vi "SLSC Convert Items - Variant to String.vi"(0 "Datatype":string, 1 "format string":string="%#_12g", 5 "value":variant, 7 "min":variant, 9 "max":variant, 11 "reset value":variant, 12 "Enum string":cluster{"name":string, "enum":string}[](array[cluster])) -> (3 "string data reset value":string, 4 "Output data type":string, 6 "string data value":string, 8 "string min":string, 10 "string max":string, 13 "Option":string, 14 "enum_range":string)   [LabVIEW 2019, in "SLSC Tree Control.lvlib"]
doc: "Converts all of the item elements from variant into strings."
uses:
  SLSC Tree Control.lvlib
  <vilib>/Utility/Data Type/Type Definitions/Data Type.ctl
  <vilib>/regexp/Match Regular Expression.xnode
  <vilib>/Utility/Data Type/NI_Data Type.lvlib
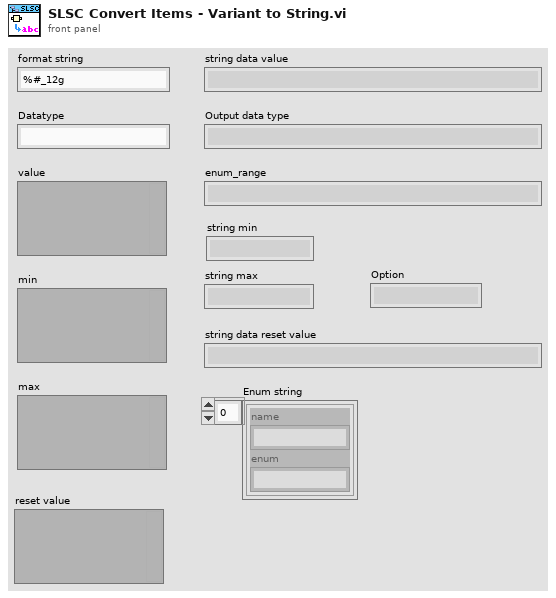
[diagram p1: front panel]
types:
  T1 = typedef "NI_Data Type.lvlib/Data Type.ctl" = enum8{"Invalid Type", "Void", "I8", "I16", "I32", "I64", "U8", "U16", "U32", "U64", "Single Float", "Double Float", "Extended Float", "Single Complex", "Double Complex", "Extended Complex", "Enum U8", "Enum U16", "Enum U32", "Enum U64", "Single Float With Unit", "Double Float With Unit", "Extended Float With Unit", "Single Complex with Unit", "Double Complex with Unit", "Extended Complex with Unit", "Boolean", "String", "Path", "Picture", "Tag", "Array", "Cluster", "Variant", "LV Variant", "Waveform", "Timestamp", "Digital Waveform", "Digital Data", "ExpressData", "Refnum", "External Data", "VI", "Poly VI", "LabVIEW Class Instance", "Fixed Point", "Set Collection", "Map Collection"}
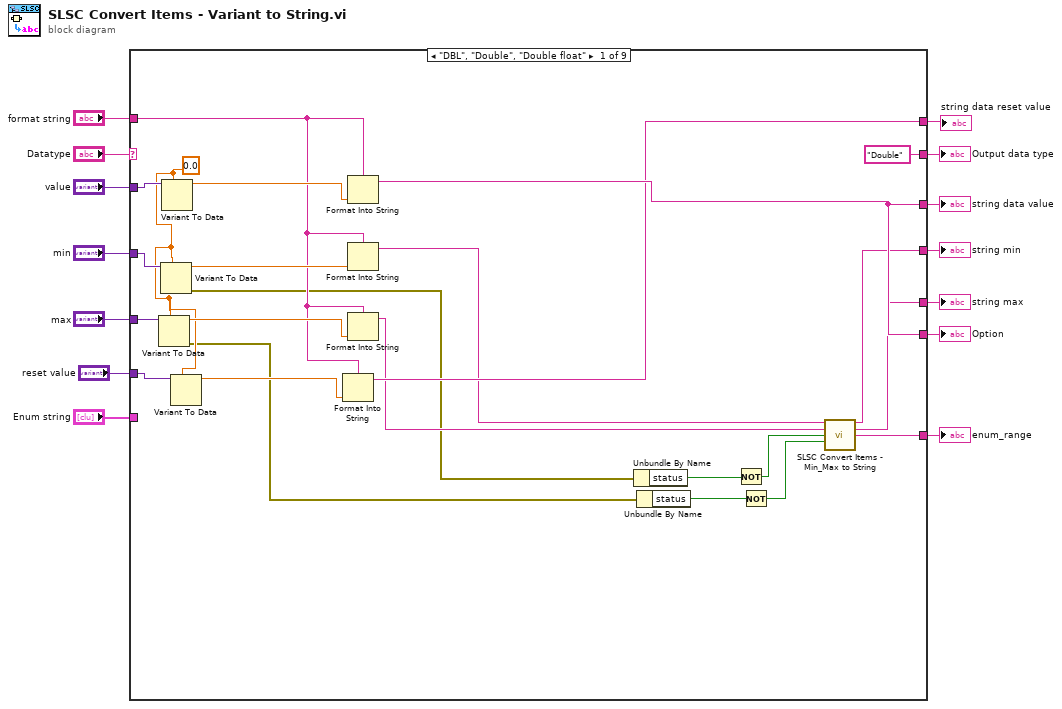
[diagram p0: block diagram]
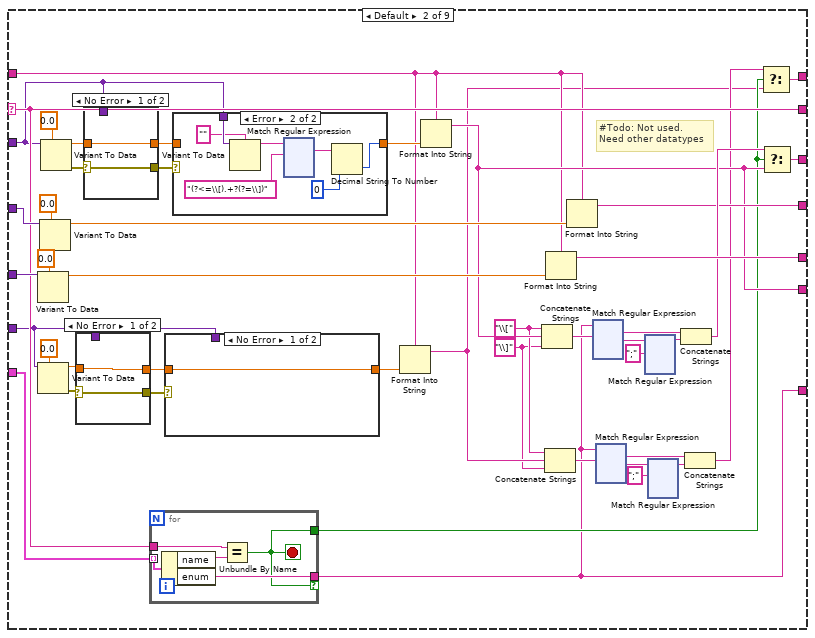
[diagram p2: hidden frame]
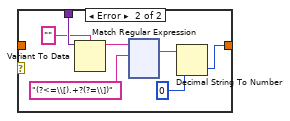
[diagram p3: hidden frame]
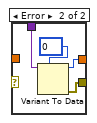
[diagram p4: hidden frame]
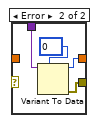
[diagram p6: hidden frame]
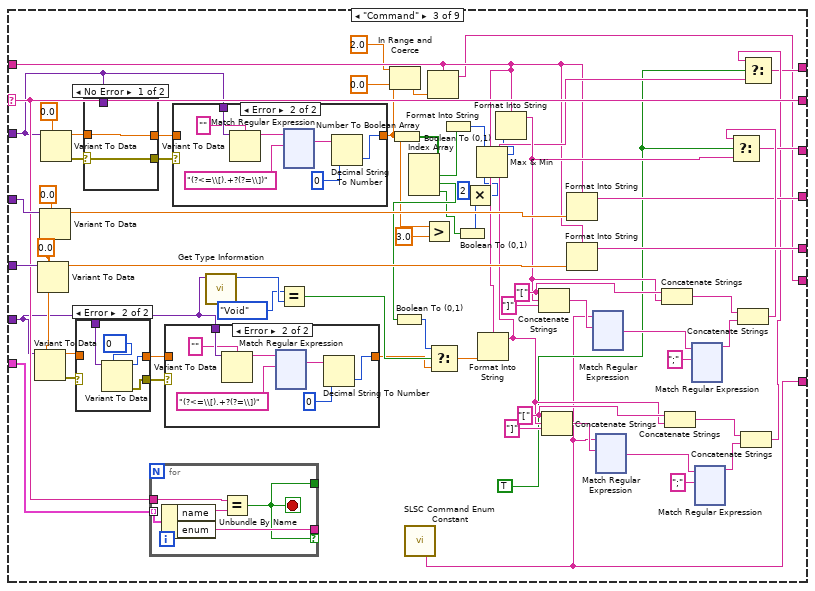
[diagram p7: hidden frame]
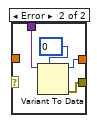
[diagram p11: hidden frame]
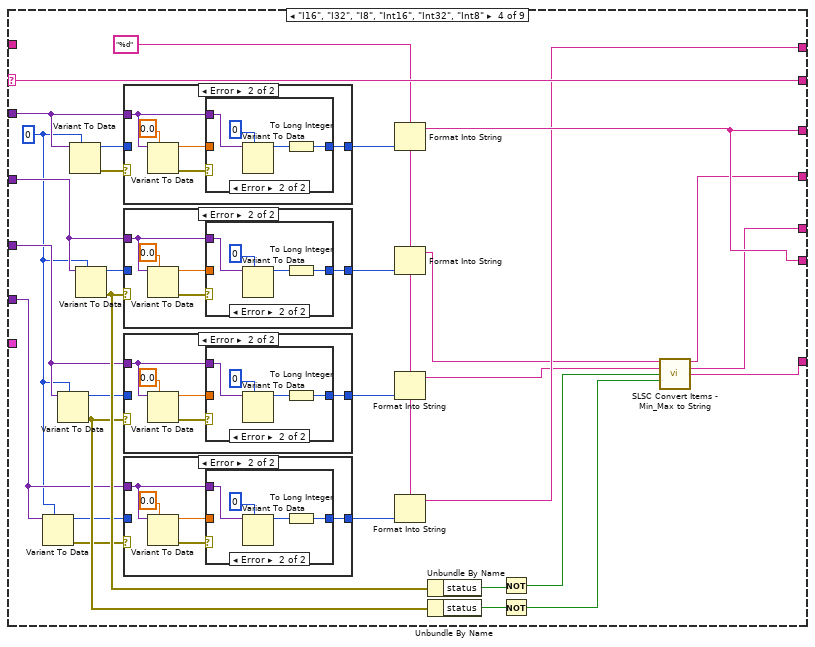
[diagram p12: hidden frame]
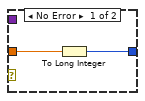
[diagram p14: hidden frame]
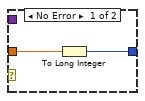
[diagram p16: hidden frame]
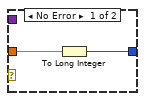
[diagram p18: hidden frame]
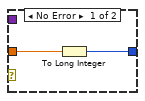
[diagram p20: hidden frame]
diagram:
  n1 = case shown="\"DBL\", \"Double\", \"Double float\"" "Datatype" {
    selector: "Datatype" -> [_ w75 w857 w1612 w1690 w1764 w1872 w1970 w2017]
    tunnel: "value" -> [w38 w63 w842 w1597 w1675 w1752 w1860 w1966 w2016]
    tunnel: [w32 w69 w848 w1611 w1689 w1763 w1871 w1971 w2015] -> w3
    tunnel: ["Double" w75 w857 w1612 w1690 w1764 w1872 w1970 w2017] -> w10
    tunnel: "min" -> [w36 w81 w863 w1595 w1673 w1745 w1857 _ _]
    tunnel: "max" -> [w35 w80 w862 w1591 w1669 w1746 w1853 _ _]
    tunnel: [w17 w66 w845 w1602 w1680 w1756 w1864 _ _] -> w6
    tunnel: [w16 w77 w859 w1601 w1679 w1755 w1863 _ _] -> w5
    tunnel: "format string" -> [w27 w53 w813 _ _ _ _ _ _]
    tunnel: "Enum string" -> [_ w76 w858 _ _ _ _ _ _]
    tunnel: [w18 w44 w816 w1603 w1681 w1757 w1865 _ _] -> w14
    tunnel: [w32 w65 w812 w1611 w1689 w1763 w1871 w1967 _] -> w4
    tunnel: "reset value" -> [w31 w54 w821 w1587 w1665 w1747 w1848 w1959 w2013]
    tunnel: [w28 w45 w826 w1610 w1688 w1762 w1870 w1955 w2012] -> w1
    frame "DBL", "Double", "Double float" {
      w30 = 0.0
      n2 = Variant To Data(type=w30, Variant=w35) -> (data=w33:dbl, error out=w23:errorcluster)  [unwired: 1 in]
      n3 = Variant To Data(type=w30, Variant=w36) -> (data=w34:dbl, error out=w24:errorcluster)  [unwired: 1 in]
      n4 = Variant To Data(type=w30, Variant=w38) -> (data=w37:dbl)  [unwired: 1 in, 1 out]
      n5 = Variant To Data(type=w30, Variant=w31) -> (data=w29:dbl)  [unwired: 1 in, 1 out]
      n6 = Format Into String(format string=w27, w29) -> (resulting string=w28:string)  [unwired: 2 in, 1 out]
      n7 = Format Into String(format string=w27, w37) -> (resulting string=w32:string)  [unwired: 2 in, 1 out]
      n8 = Format Into String(format string=w27, w34) -> (resulting string=w26:string)  [unwired: 2 in, 1 out]
      n9 = Format Into String(format string=w27, w33) -> (resulting string=w25:string)  [unwired: 2 in, 1 out]
      n10 = Unbundle By Name(w24) -> ("status"=w21:bool)
      n11 = Unbundle By Name(w23) -> ("status"=w22:bool)
      n12 = Not(x=w21) -> (.not. x?=w19:bool)
      n13 = Not(x=w22) -> (.not. x?=w20:bool)
      n14 = call "SLSC Convert Items - Min_Max to String.vi"("minimum"=w26, "maximum"=w25, "min?"=w19, "max?"=w20) -> ("minimum out"=w17:string, "maximum out"=w16:string, "minmax string"=w18:string)  [unwired: 9 in]
    }
    frame Default {
      w42 = "\\]" ("string")
      w43 = "\\[" ("string")
      # "#Todo: Not used.\nNeed other datatypes"
      n15 = Variant To Data(type=0.0, Variant=w80) -> (data=w78:dbl)  [unwired: 1 in, 1 out]
      n16 = Variant To Data(type=0.0, Variant=w54) -> (data=w56:dbl, error out=w57:errorcluster)  [unwired: 1 in]
      n17 = Variant To Data(type=0.0, Variant=w81) -> (data=w79:dbl)  [unwired: 1 in, 1 out]
      n18 = Variant To Data(type=0.0, Variant=w63) -> (data=w67:dbl, error out=w68:errorcluster)  [unwired: 1 in]
      n19 = case shown="No Error" w57 {
        selector: w57 -> [w434 _]
        tunnel: w54 -> [_ w439]
        tunnel: [w435 w438] -> w58
        tunnel: w56 -> [w435 _]
        tunnel: [w434 w436] -> w59
        frame No Error {
        }
        frame Error {
          w437 = u16 0 items=[""] ("Ring")
          n20 = Variant To Data(type=w437, Variant=w439) -> (data=w438:u16, error out=w436:errorcluster)  [unwired: 1 in]
        }
      }
      n21 = case shown="No Error" w68 {
        selector: w68 -> [w562 _]
        tunnel: w63 -> [_ w567]
        tunnel: [w563 w566] -> w64
        tunnel: w67 -> [w563 _]
        tunnel: [w562 w564] -> w62
        frame No Error {
        }
        frame Error {
          w565 = u16 0 items=[""] ("Ring")
          n22 = Variant To Data(type=w565, Variant=w567) -> (data=w566:u16, error out=w564:errorcluster)  [unwired: 1 in]
        }
      }
      n23 = for {
        tunnel: w76 -> [w800] mode=indexing
        tunnel: w75 -> [w798]
        tunnel: [w797] -> w44 if=w796
        tunnel: [w796] -> w48
        stop <- w796 stop-if-true
        n24 = Unbundle By Name(w800) -> ("name"=w799:string, "enum"=w797:string)
        n25 = Equal?(x=w798, y=w799) -> (x = y?=w796:bool)
      }
      n26 = case shown="No Error" w59 {
        tunnel: w54 -> [_ w319]
        tunnel: [w312 w313] -> w60
        tunnel: w58 -> [w312 _]
        frame No Error {
        }
        frame Error {
          n27 = Variant To Data(type="", Variant=w319) -> (data=w317:string)  [unwired: 1 in, 1 out]
          n28 = xnode "Match Regular Expression"("input string"=w317, "regular expression"="(?<=\\[).+?(?=\\])") -> ("whole match"=w315:string)  [unwired: 4 in, 4 out]
          n29 = Decimal String To Number(string=w315, default (0L)=0) -> (number=w313:i32)  [unwired: 1 in, 1 out]
        }
      }
      n30 = case shown="Error" w62 {
        tunnel: w63 -> [_ w447]
        tunnel: [w440 w441] -> w61
        tunnel: w64 -> [w440 _]
        frame No Error {
        }
        frame Error {
          n31 = Variant To Data(type="", Variant=w447) -> (data=w445:string)  [unwired: 1 in, 1 out]
          n32 = xnode "Match Regular Expression"("input string"=w445, "regular expression"="(?<=\\[).+?(?=\\])") -> ("whole match"=w443:string)  [unwired: 4 in, 4 out]
          n33 = Decimal String To Number(string=w443, default (0L)=0) -> (number=w441:i32)  [unwired: 1 in, 1 out]
        }
      }
      n34 = Format Into String(format string=w53, w60) -> (resulting string=w46:string)  [unwired: 2 in, 1 out]
      n35 = Format Into String(format string=w53, w61) -> (resulting string=w65:string)  [unwired: 2 in, 1 out]
      n36 = Concatenate Strings(w43, w65, w42) -> (w71:string)
      n37 = Concatenate Strings(w43, w46, w42) -> (w52:string)
      n38 = Format Into String(format string=w53, w78) -> (resulting string=w77:string)  [unwired: 2 in, 1 out]
      n39 = Format Into String(format string=w53, w79) -> (resulting string=w66:string)  [unwired: 2 in, 1 out]
      n40 = xnode "Match Regular Expression"("input string"=w44, "regular expression"=w71) -> ("whole match"=w41:string, "after match"=w74:string)  [unwired: 4 in, 3 out]
      n41 = xnode "Match Regular Expression"("input string"=w44, "regular expression"=w52) -> ("whole match"=w40:string, "after match"=w49:string)  [unwired: 4 in, 3 out]
      n42 = xnode "Match Regular Expression"("input string"=w74, "regular expression"=";") -> ("before match"=w72:string)  [unwired: 4 in, 4 out]
      n43 = xnode "Match Regular Expression"("input string"=w49, "regular expression"=";") -> ("before match"=w51:string)  [unwired: 4 in, 4 out]
      n44 = Concatenate Strings(w41, w72) -> (w70:string)
      n45 = Concatenate Strings(w40, w51) -> (w47:string)
      n46 = Select(t=w47, s=w48, f=w46) -> (s? t:f=w45:string)
      n47 = Select(t=w70, s=w48, f=w65) -> (s? t:f=w69:string)
    }
    frame "Command" {
      w825 = TRUE ("s")
      w834 = "[" ("string")
      w851 = "[" ("string")
      w836 = 0.0
      n48 = Variant To Data(type=w836, Variant=w821) -> (data=w837:dbl, error out=w838:errorcluster)  [unwired: 1 in]
      n49 = Variant To Data(type=w836, Variant=w862) -> (data=w860:dbl)  [unwired: 1 in, 1 out]
      n50 = Variant To Data(type=0.0, Variant=w863) -> (data=w861:dbl)  [unwired: 1 in, 1 out]
      n51 = Variant To Data(type=0.0, Variant=w842) -> (data=w846:dbl, error out=w847:errorcluster)  [unwired: 1 in]
      n52 = case shown="Error" w838 {
        selector: w838 -> [w1216 _]
        tunnel: w821 -> [_ w1221]
        tunnel: [w1217 w1220] -> w839
        tunnel: w837 -> [w1217 _]
        tunnel: [w1216 w1218] -> w840
        frame No Error {
        }
        frame Error {
          w1219 = u16 0 items=[""] ("Ring")
          n53 = Variant To Data(type=w1219, Variant=w1221) -> (data=w1220:u16, error out=w1218:errorcluster)  [unwired: 1 in]
        }
      }
      n54 = case shown="No Error" w847 {
        selector: w847 -> [w1344 _]
        tunnel: w842 -> [_ w1349]
        tunnel: [w1345 w1348] -> w843
        tunnel: w846 -> [w1345 _]
        tunnel: [w1344 w1346] -> w841
        frame No Error {
        }
        frame Error {
          w1347 = u16 0 items=[""] ("Ring")
          n55 = Variant To Data(type=w1347, Variant=w1349) -> (data=w1348:u16, error out=w1346:errorcluster)  [unwired: 1 in]
        }
      }
      n56 = for {
        tunnel: w858 -> [w1582] mode=indexing
        tunnel: w857 -> [w1580]
        tunnel: [w1579] -> _ if=w1578
        tunnel: [w1578] -> _
        stop <- w1578 stop-if-true
        n57 = Unbundle By Name(w1582) -> ("name"=w1581:string, "enum"=w1579:string)
        n58 = Equal?(x=w1580, y=w1581) -> (x = y?=w1578:bool)
      }
      n59 = case shown="Error" w840 {
        tunnel: w821 -> [_ w1101]
        tunnel: [w1094 w1095] -> w815
        tunnel: w839 -> [w1094 _]
        frame No Error {
        }
        frame Error {
          n60 = Variant To Data(type="", Variant=w1101) -> (data=w1099:string)  [unwired: 1 in, 1 out]
          n61 = xnode "Match Regular Expression"("input string"=w1099, "regular expression"="(?<=\\[).+?(?=\\])") -> ("whole match"=w1097:string)  [unwired: 4 in, 4 out]
          n62 = Decimal String To Number(string=w1097, default (0L)=0) -> (number=w1095:i32)  [unwired: 1 in, 1 out]
        }
      }
      n63 = case shown="Error" w841 {
        tunnel: w842 -> [_ w1229]
        tunnel: [w1222 w1223] -> w811
        tunnel: w843 -> [w1222 _]
        frame No Error {
        }
        frame Error {
          n64 = Variant To Data(type="", Variant=w1229) -> (data=w1227:string)  [unwired: 1 in, 1 out]
          n65 = xnode "Match Regular Expression"("input string"=w1227, "regular expression"="(?<=\\[).+?(?=\\])") -> ("whole match"=w1225:string)  [unwired: 4 in, 4 out]
          n66 = Decimal String To Number(string=w1225, default (0L)=0) -> (number=w1223:i32)  [unwired: 1 in, 1 out]
        }
      }
      n67 = call <vilib>:"Get Type Information.vi"("variant"=w821) -> ("type"=w820:T1)  [unwired: 6 in, 4 out]
      n68 = Equal?(x=Data_Type."Void", y=w820) -> (x = y?=w818:bool)
      n69 = In Range and Coerce(upper limit=2.0 ("x"), x=w811, lower limit=0.0 ("x")) -> (coerced(x)=w807:dbl)  [unwired: 1 out]
      n70 = Number To Boolean Array(number=w811) -> (Boolean array=w824:bool[])
      n71 = call "SLSC Command Enum Constant.vi"() -> ("string enums"=w816:string)  [unwired: 11 in, 4 out]
      n72 = Index Array(array=w824) -> (element #1=w823:bool, element #2=w822:bool, element #3=w804:bool)  [unwired: 3 in]
      n73 = Boolean To (0,1)(Boolean=w822) -> (0, 1=w817:i16)
      n74 = Greater?(x=w811, y=3.0) -> ()  [unwired: 1 out]
      n75 = Format Into String(format string=w813, w807) -> (resulting string=w812:string)  [unwired: 2 in, 1 out]
      n76 = Select(t=w817, s=w818, f=w815) -> (s? t:f=w814:dbl)
      n77 = Boolean To (0,1)(Boolean=w823) -> (0, 1=w802:i16)
      n78 = Boolean To (0,1)(Boolean=w804) -> (0, 1=w809:i16)
      n79 = Multiply(x=i16 2, y=w809) -> (x*y=w803:i16)
      n80 = Max & Min(x=w802, y=w803) -> (max(x,y)=w801:i16)  [unwired: 1 out]
      n81 = Format Into String(format string=w813, w814) -> (resulting string=w827:string)  [unwired: 2 in, 1 out]
      n82 = Format Into String(format string=w813, w801) -> (resulting string=w844:string)  [unwired: 2 in, 1 out]
      n83 = Concatenate Strings(w851, w844, "]" ("string")) -> (w852:string)
      n84 = Concatenate Strings(w834, w827, "]" ("string")) -> (w833:string)
      n85 = Format Into String(format string=w813, w861) -> (resulting string=w845:string)  [unwired: 2 in, 1 out]
      n86 = Format Into String(format string=w813, w860) -> (resulting string=w859:string)  [unwired: 2 in, 1 out]
      n87 = xnode "Match Regular Expression"("input string"=w816, "regular expression"=w852) -> ("after match"=w855:string)  [unwired: 4 in, 4 out]
      n88 = xnode "Match Regular Expression"("input string"=w816, "regular expression"=w833) -> ("after match"=w830:string)  [unwired: 4 in, 4 out]
      n89 = Concatenate Strings(w851, w844) -> (w850:string)
      n90 = Concatenate Strings(w834, w827) -> (w835:string)
      n91 = xnode "Match Regular Expression"("input string"=w855, "regular expression"=";") -> ("before match"=w853:string)  [unwired: 4 in, 4 out]
      n92 = xnode "Match Regular Expression"("input string"=w830, "regular expression"=";") -> ("before match"=w832:string)  [unwired: 4 in, 4 out]
      n93 = Concatenate Strings(w850, w853) -> (w849:string)
      n94 = Select(t=w849, s=w825, f=w844) -> (s? t:f=w848:string)
      n95 = Concatenate Strings(w835, w832) -> (w828:string)
      n96 = Select(t=w828, s=w825, f=w827) -> (s? t:f=w826:string)
    }
    frame "I16", "I32", "I8", "Int16", "Int32", "Int8" {
      w1583 = 0
      w1600 = "%d" ("format string")
      n97 = Variant To Data(type=w1583, Variant=w1587) -> (data=w1585:i32, error out=w1586:errorcluster)  [unwired: 1 in]
      n98 = Variant To Data(type=w1583, Variant=w1591) -> (data=w1588:i32, error out=w1589:errorcluster)  [unwired: 1 in]
      n99 = Variant To Data(type=w1583, Variant=w1597) -> (data=w1599:i32, error out=w1598:errorcluster)  [unwired: 1 in]
      n100 = Variant To Data(type=w1583, Variant=w1595) -> (data=w1594:i32, error out=w1593:errorcluster)  [unwired: 1 in]
      n101 = case shown="Error" w1598 {
        tunnel: [w1649 w1651] -> w1596
        tunnel: w1599 -> [w1649 _]
        tunnel: w1597 -> [_ w1653]
        frame No Error {
        }
        frame Error {
          n102 = Variant To Data(type=0.0, Variant=w1653) -> (data=w1650:dbl, error out=w1652:errorcluster)  [unwired: 1 in]
          n103 = case shown="Error" w1652 {
            tunnel: w1653 -> [_ w1659]
            tunnel: [w1655 w1657] -> w1651
            tunnel: w1650 -> [w1656 _]
            frame No Error {
              n104 = To Long Integer(number=w1656) -> (32bit integer=w1655:i32)
            }
            frame Error {
              n105 = Variant To Data(type=i16 0, Variant=w1659) -> (data=w1658:i16)  [unwired: 1 in, 1 out]
              n106 = To Long Integer(number=w1658) -> (32bit integer=w1657:i32)
            }
          }
        }
      }
      n107 = case shown="Error" w1593 {
        tunnel: [w1637 w1639] -> w1592
        tunnel: w1594 -> [w1637 _]
        tunnel: w1595 -> [_ w1641]
        frame No Error {
        }
        frame Error {
          n108 = Variant To Data(type=0.0, Variant=w1641) -> (data=w1638:dbl, error out=w1640:errorcluster)  [unwired: 1 in]
          n109 = case shown="Error" w1640 {
            tunnel: w1641 -> [_ w1647]
            tunnel: [w1643 w1645] -> w1639
            tunnel: w1638 -> [w1644 _]
            frame No Error {
              n110 = To Long Integer(number=w1644) -> (32bit integer=w1643:i32)
            }
            frame Error {
              n111 = Variant To Data(type=i16 0, Variant=w1647) -> (data=w1646:i16)  [unwired: 1 in, 1 out]
              n112 = To Long Integer(number=w1646) -> (32bit integer=w1645:i32)
            }
          }
        }
      }
      n113 = case shown="Error" w1589 {
        tunnel: [w1625 w1627] -> w1590
        tunnel: w1588 -> [w1625 _]
        tunnel: w1591 -> [_ w1629]
        frame No Error {
        }
        frame Error {
          n114 = Variant To Data(type=0.0, Variant=w1629) -> (data=w1626:dbl, error out=w1628:errorcluster)  [unwired: 1 in]
          n115 = case shown="Error" w1628 {
            tunnel: w1629 -> [_ w1635]
            tunnel: [w1631 w1633] -> w1627
            tunnel: w1626 -> [w1632 _]
            frame No Error {
              n116 = To Long Integer(number=w1632) -> (32bit integer=w1631:i32)
            }
            frame Error {
              n117 = Variant To Data(type=i16 0, Variant=w1635) -> (data=w1634:i16)  [unwired: 1 in, 1 out]
              n118 = To Long Integer(number=w1634) -> (32bit integer=w1633:i32)
            }
          }
        }
      }
      n119 = case shown="Error" w1586 {
        tunnel: [w1613 w1615] -> w1584
        tunnel: w1585 -> [w1613 _]
        tunnel: w1587 -> [_ w1617]
        frame No Error {
        }
        frame Error {
          n120 = Variant To Data(type=0.0, Variant=w1617) -> (data=w1614:dbl, error out=w1616:errorcluster)  [unwired: 1 in]
          n121 = case shown="Error" w1616 {
            tunnel: w1617 -> [_ w1623]
            tunnel: [w1619 w1621] -> w1615
            tunnel: w1614 -> [w1620 _]
            frame No Error {
              n122 = To Long Integer(number=w1620) -> (32bit integer=w1619:i32)
            }
            frame Error {
              n123 = Variant To Data(type=i16 0, Variant=w1623) -> (data=w1622:i16)  [unwired: 1 in, 1 out]
              n124 = To Long Integer(number=w1622) -> (32bit integer=w1621:i32)
            }
          }
        }
      }
      n125 = Format Into String(format string=w1600, w1596) -> (resulting string=w1611:string)  [unwired: 2 in, 1 out]
      n126 = Format Into String(format string=w1600, w1592) -> (resulting string=w1605:string)  [unwired: 2 in, 1 out]
      n127 = Format Into String(format string=w1600, w1590) -> (resulting string=w1604:string)  [unwired: 2 in, 1 out]
      n128 = Format Into String(format string=w1600, w1584) -> (resulting string=w1610:string)  [unwired: 2 in, 1 out]
      n129 = Unbundle By Name(w1593) -> ("status"=w1608:bool)
      n130 = Unbundle By Name(w1589) -> ("status"=w1609:bool)
      n131 = Not(x=w1608) -> (.not. x?=w1606:bool)
      n132 = Not(x=w1609) -> (.not. x?=w1607:bool)
      n133 = call "SLSC Convert Items - Min_Max to String.vi"("minimum"=w1605, "maximum"=w1604, "min?"=w1606, "max?"=w1607) -> ("minimum out"=w1602:string, "maximum out"=w1601:string, "minmax string"=w1603:string)  [unwired: 9 in]
    }
    frame "U16", "U32", "U8", "UInt16", "UInt32", "UInt8" {
      w1661 = u32 0
      w1678 = "%d" ("format string")
      n134 = Variant To Data(type=w1661, Variant=w1665) -> (data=w1663:u32, error out=w1664:errorcluster)  [unwired: 1 in]
      n135 = Variant To Data(type=w1661, Variant=w1669) -> (data=w1666:u32, error out=w1667:errorcluster)  [unwired: 1 in]
      n136 = Variant To Data(type=w1661, Variant=w1675) -> (data=w1677:u32, error out=w1676:errorcluster)  [unwired: 1 in]
      n137 = Variant To Data(type=w1661, Variant=w1673) -> (data=w1672:u32, error out=w1671:errorcluster)  [unwired: 1 in]
      n138 = case shown="Error" w1676 {
        tunnel: [w1727 w1729] -> w1674
        tunnel: w1677 -> [w1727 _]
        tunnel: w1675 -> [_ w1731]
        frame No Error {
        }
        frame Error {
          n139 = Variant To Data(type=0.0, Variant=w1731) -> (data=w1728:dbl, error out=w1730:errorcluster)  [unwired: 1 in]
          n140 = case shown="Error" w1730 {
            tunnel: w1731 -> [_ w1737]
            tunnel: [w1733 w1735] -> w1729
            tunnel: w1728 -> [w1734 _]
            frame No Error {
              n141 = To Long Integer(number=w1734) -> (32bit integer=w1733:i32)
            }
            frame Error {
              n142 = Variant To Data(type=u16 0, Variant=w1737) -> (data=w1736:u16)  [unwired: 1 in, 1 out]
              n143 = To Unsigned Long Integer(number=w1736) -> (unsigned 32bit integer=w1735:u32)
            }
          }
        }
      }
      n144 = case shown="Error" w1671 {
        tunnel: [w1715 w1717] -> w1670
        tunnel: w1672 -> [w1715 _]
        tunnel: w1673 -> [_ w1719]
        frame No Error {
        }
        frame Error {
          n145 = Variant To Data(type=0.0, Variant=w1719) -> (data=w1716:dbl, error out=w1718:errorcluster)  [unwired: 1 in]
          n146 = case shown="Error" w1718 {
            tunnel: w1719 -> [_ w1725]
            tunnel: [w1721 w1723] -> w1717
            tunnel: w1716 -> [w1722 _]
            frame No Error {
              n147 = To Long Integer(number=w1722) -> (32bit integer=w1721:i32)
            }
            frame Error {
              n148 = Variant To Data(type=u16 0, Variant=w1725) -> (data=w1724:u16)  [unwired: 1 in, 1 out]
              n149 = To Unsigned Long Integer(number=w1724) -> (unsigned 32bit integer=w1723:u32)
            }
          }
        }
      }
      n150 = case shown="Error" w1667 {
        tunnel: [w1703 w1705] -> w1668
        tunnel: w1666 -> [w1703 _]
        tunnel: w1669 -> [_ w1707]
        frame No Error {
        }
        frame Error {
          n151 = Variant To Data(type=0.0, Variant=w1707) -> (data=w1704:dbl, error out=w1706:errorcluster)  [unwired: 1 in]
          n152 = case shown="Error" w1706 {
            tunnel: w1707 -> [_ w1713]
            tunnel: [w1709 w1711] -> w1705
            tunnel: w1704 -> [w1710 _]
            frame No Error {
              n153 = To Long Integer(number=w1710) -> (32bit integer=w1709:i32)
            }
            frame Error {
              n154 = Variant To Data(type=u16 0, Variant=w1713) -> (data=w1712:u16)  [unwired: 1 in, 1 out]
              n155 = To Unsigned Long Integer(number=w1712) -> (unsigned 32bit integer=w1711:u32)
            }
          }
        }
      }
      n156 = case shown="Error" w1664 {
        tunnel: [w1691 w1693] -> w1662
        tunnel: w1663 -> [w1691 _]
        tunnel: w1665 -> [_ w1695]
        frame No Error {
        }
        frame Error {
          n157 = Variant To Data(type=0.0, Variant=w1695) -> (data=w1692:dbl, error out=w1694:errorcluster)  [unwired: 1 in]
          n158 = case shown="Error" w1694 {
            tunnel: w1695 -> [_ w1701]
            tunnel: [w1697 w1699] -> w1693
            tunnel: w1692 -> [w1698 _]
            frame No Error {
              n159 = To Long Integer(number=w1698) -> (32bit integer=w1697:i32)
            }
            frame Error {
              n160 = Variant To Data(type=u16 0, Variant=w1701) -> (data=w1700:u16)  [unwired: 1 in, 1 out]
              n161 = To Unsigned Long Integer(number=w1700) -> (unsigned 32bit integer=w1699:u32)
            }
          }
        }
      }
      n162 = Format Into String(format string=w1678, w1674) -> (resulting string=w1689:string)  [unwired: 2 in, 1 out]
      n163 = Format Into String(format string=w1678, w1670) -> (resulting string=w1683:string)  [unwired: 2 in, 1 out]
      n164 = Format Into String(format string=w1678, w1668) -> (resulting string=w1682:string)  [unwired: 2 in, 1 out]
      n165 = Format Into String(format string=w1678, w1662) -> (resulting string=w1688:string)  [unwired: 2 in, 1 out]
      n166 = Unbundle By Name(w1671) -> ("status"=w1686:bool)
      n167 = Unbundle By Name(w1667) -> ("status"=w1687:bool)
      n168 = Not(x=w1686) -> (.not. x?=w1684:bool)
      n169 = Not(x=w1687) -> (.not. x?=w1685:bool)
      n170 = call "SLSC Convert Items - Min_Max to String.vi"("minimum"=w1683, "maximum"=w1682, "min?"=w1684, "max?"=w1685) -> ("minimum out"=w1680:string, "maximum out"=w1679:string, "minmax string"=w1681:string)  [unwired: 9 in]
    }
    frame "U64", "Uint64" {
      w1739 = u64 0
      w1754 = "%d" ("format string")
      n171 = call <vilib>:"Get Type Information.vi"("variant"=w1752) -> ("type"=w1751:T1)  [unwired: 6 in, 4 out]
      n172 = call <vilib>:"Get Type Information.vi"("variant"=w1747) -> ("type"=w1748:T1)  [unwired: 6 in, 4 out]
      n173 = call <vilib>:"Get Type Information.vi"("variant"=w1745) -> ("type"=w1750:T1)  [unwired: 6 in, 4 out]
      n174 = call <vilib>:"Get Type Information.vi"("variant"=w1746) -> ("type"=w1749:T1)  [unwired: 6 in, 4 out]
      n175 = case shown="\"U32\"" w1751 {
        tunnel: [_ w1828 w1830 w1834 w1838 w1843] -> w1753
        tunnel: w1752 -> [_ w1829 w1833 w1837 w1841 w1845]
        tunnel: w1739 -> [_ w1827 _ _ _ w1842]
        frame "Invalid Type", "Void", Default {
        }
        frame "U64" {
          n176 = Variant To Data(type=w1827, Variant=w1829) -> (data=w1828:u64)  [unwired: 1 in, 1 out]
        }
        frame "U32" {
          n177 = Variant To Data(type=u32 0, Variant=w1833) -> (data=w1832:u32)  [unwired: 1 in, 1 out]
          n178 = To Unsigned Quad Integer(1:w1832) -> (0:w1830:u64)
        }
        frame "U16" {
          n179 = Variant To Data(type=u16 0, Variant=w1837) -> (data=w1836:u16)  [unwired: 1 in, 1 out]
          n180 = To Unsigned Quad Integer(1:w1836) -> (0:w1834:u64)
        }
        frame "U8" {
          n181 = Variant To Data(type=u8 0, Variant=w1841) -> (data=w1840:u8)  [unwired: 1 in, 1 out]
          n182 = To Unsigned Quad Integer(1:w1840) -> (0:w1838:u64)
        }
        frame "Double Float" {
          n183 = Variant To Data(type=0.0, Variant=w1845) -> (data=w1844:dbl)  [unwired: 1 in, 1 out]
          n184 = Type Cast(type=w1842, x=w1844) -> (*(type *) &x=w1843:u64)
        }
      }
      n185 = case shown="\"Double Float\"" w1748 {
        tunnel: [_ w1766 w1768 w1772 w1776 w1781] -> w1742
        tunnel: w1747 -> [_ w1767 w1771 w1775 w1779 w1783]
        tunnel: w1739 -> [_ w1765 _ _ _ w1780]
        frame "Invalid Type", "Void", Default {
        }
        frame "U64" {
          n186 = Variant To Data(type=w1765, Variant=w1767) -> (data=w1766:u64)  [unwired: 1 in, 1 out]
        }
        frame "U32" {
          n187 = Variant To Data(type=u32 0, Variant=w1771) -> (data=w1770:u32)  [unwired: 1 in, 1 out]
          n188 = To Unsigned Quad Integer(1:w1770) -> (0:w1768:u64)
        }
        frame "U16" {
          n189 = Variant To Data(type=u16 0, Variant=w1775) -> (data=w1774:u16)  [unwired: 1 in, 1 out]
          n190 = To Unsigned Quad Integer(1:w1774) -> (0:w1772:u64)
        }
        frame "U8" {
          n191 = Variant To Data(type=u8 0, Variant=w1779) -> (data=w1778:u8)  [unwired: 1 in, 1 out]
          n192 = To Unsigned Quad Integer(1:w1778) -> (0:w1776:u64)
        }
        frame "Double Float" {
          n193 = Variant To Data(type=0.0, Variant=w1783) -> (data=w1782:dbl)  [unwired: 1 in, 1 out]
          n194 = Type Cast(type=w1780, x=w1782) -> (*(type *) &x=w1781:u64)
        }
      }
      n195 = case shown="\"U64\"" w1750 {
        tunnel: [_ w1808 w1810 w1814 w1818 w1823] -> w1744
        tunnel: w1745 -> [_ w1809 w1813 w1817 w1821 w1825]
        tunnel: [TRUE _ _ _ _ _] -> w1741
        tunnel: w1739 -> [_ w1807 _ _ _ w1822]
        frame "Invalid Type", "Void", Default {
        }
        frame "U64" {
          n196 = Variant To Data(type=w1807, Variant=w1809) -> (data=w1808:u64)  [unwired: 1 in, 1 out]
        }
        frame "U32" {
          n197 = Variant To Data(type=u32 0, Variant=w1813) -> (data=w1812:u32)  [unwired: 1 in, 1 out]
          n198 = To Unsigned Quad Integer(1:w1812) -> (0:w1810:u64)
        }
        frame "U16" {
          n199 = Variant To Data(type=u16 0, Variant=w1817) -> (data=w1816:u16)  [unwired: 1 in, 1 out]
          n200 = To Unsigned Quad Integer(1:w1816) -> (0:w1814:u64)
        }
        frame "U8" {
          n201 = Variant To Data(type=u8 0, Variant=w1821) -> (data=w1820:u8)  [unwired: 1 in, 1 out]
          n202 = To Unsigned Quad Integer(1:w1820) -> (0:w1818:u64)
        }
        frame "Double Float" {
          n203 = Variant To Data(type=0.0, Variant=w1825) -> (data=w1824:dbl)  [unwired: 1 in, 1 out]
          n204 = Type Cast(type=w1822, x=w1824) -> (*(type *) &x=w1823:u64)
        }
      }
      n205 = case shown="\"Double Float\"" w1749 {
        tunnel: [_ w1787 w1789 w1793 w1797 w1802] -> w1743
        tunnel: w1746 -> [_ w1788 w1792 w1796 w1800 w1804]
        tunnel: [TRUE _ _ _ _ _] -> w1740
        tunnel: w1739 -> [_ w1786 _ _ _ w1801]
        frame "Invalid Type", "Void", Default {
        }
        frame "U64" {
          n206 = Variant To Data(type=w1786, Variant=w1788) -> (data=w1787:u64)  [unwired: 1 in, 1 out]
        }
        frame "U32" {
          n207 = Variant To Data(type=u32 0, Variant=w1792) -> (data=w1791:u32)  [unwired: 1 in, 1 out]
          n208 = To Unsigned Quad Integer(1:w1791) -> (0:w1789:u64)
        }
        frame "U16" {
          n209 = Variant To Data(type=u16 0, Variant=w1796) -> (data=w1795:u16)  [unwired: 1 in, 1 out]
          n210 = To Unsigned Quad Integer(1:w1795) -> (0:w1793:u64)
        }
        frame "U8" {
          n211 = Variant To Data(type=u8 0, Variant=w1800) -> (data=w1799:u8)  [unwired: 1 in, 1 out]
          n212 = To Unsigned Quad Integer(1:w1799) -> (0:w1797:u64)
        }
        frame "Double Float" {
          n213 = Variant To Data(type=0.0, Variant=w1804) -> (data=w1803:dbl)  [unwired: 1 in, 1 out]
          n214 = Type Cast(type=w1801, x=w1803) -> (*(type *) &x=w1802:u64)
        }
      }
      n215 = Format Into String(format string=w1754, w1753) -> (resulting string=w1763:string)  [unwired: 2 in, 1 out]
      n216 = Format Into String(format string=w1754, w1744) -> (resulting string=w1759:string)  [unwired: 2 in, 1 out]
      n217 = Format Into String(format string=w1754, w1743) -> (resulting string=w1758:string)  [unwired: 2 in, 1 out]
      n218 = Format Into String(format string=w1754, w1742) -> (resulting string=w1762:string)  [unwired: 2 in, 1 out]
      n219 = Not(x=w1741) -> (.not. x?=w1760:bool)
      n220 = Not(x=w1740) -> (.not. x?=w1761:bool)
      n221 = call "SLSC Convert Items - Min_Max to String.vi"("minimum"=w1759, "maximum"=w1758, "min?"=w1760, "max?"=w1761) -> ("minimum out"=w1756:string, "maximum out"=w1755:string, "minmax string"=w1757:string)  [unwired: 9 in]
    }
    frame "I64", "Int64" {
      w1849 = i64 0
      w1862 = "%d" ("format string")
      n222 = call <vilib>:"Get Type Information.vi"("variant"=w1860) -> ("type"=w1859:T1)  [unwired: 6 in, 4 out]
      n223 = call <vilib>:"Get Type Information.vi"("variant"=w1848) -> ("type"=w1850:T1)  [unwired: 6 in, 4 out]
      n224 = call <vilib>:"Get Type Information.vi"("variant"=w1857) -> ("type"=w1858:T1)  [unwired: 6 in, 4 out]
      n225 = call <vilib>:"Get Type Information.vi"("variant"=w1853) -> ("type"=w1854:T1)  [unwired: 6 in, 4 out]
      n226 = case shown="\"I64\"" w1850 {
        tunnel: [_ w1874 w1876 w1880 w1884 w1889] -> w1847
        tunnel: w1848 -> [_ w1875 w1879 w1883 w1887 w1891]
        tunnel: w1849 -> [_ w1873 _ _ _ w1888]
        frame "Invalid Type", "Void", Default {
        }
        frame "I64" {
          n227 = Variant To Data(type=w1873, Variant=w1875) -> (data=w1874:i64)  [unwired: 1 in, 1 out]
        }
        frame "I32" {
          n228 = Variant To Data(type=0, Variant=w1879) -> (data=w1878:i32)  [unwired: 1 in, 1 out]
          n229 = To Quad Integer(1:w1878) -> (0:w1876:i64)
        }
        frame "I16" {
          n230 = Variant To Data(type=i16 0, Variant=w1883) -> (data=w1882:i16)  [unwired: 1 in, 1 out]
          n231 = To Quad Integer(1:w1882) -> (0:w1880:i64)
        }
        frame "I8" {
          n232 = Variant To Data(type=i8 0, Variant=w1887) -> (data=w1886:i8)  [unwired: 1 in, 1 out]
          n233 = To Quad Integer(1:w1886) -> (0:w1884:i64)
        }
        frame "Double Float" {
          n234 = Variant To Data(type=0.0, Variant=w1891) -> (data=w1890:dbl)  [unwired: 1 in, 1 out]
          n235 = Type Cast(type=w1888, x=w1890) -> (*(type *) &x=w1889:i64)
        }
      }
      n236 = case shown="\"Double Float\"" w1859 {
        tunnel: [_ w1936 w1938 w1942 w1946 w1951] -> w1861
        tunnel: w1860 -> [_ w1937 w1941 w1945 w1949 w1953]
        tunnel: w1849 -> [_ w1935 _ _ _ w1950]
        frame "Invalid Type", "Void", Default {
        }
        frame "I64" {
          n237 = Variant To Data(type=w1935, Variant=w1937) -> (data=w1936:i64)  [unwired: 1 in, 1 out]
        }
        frame "I32" {
          n238 = Variant To Data(type=0, Variant=w1941) -> (data=w1940:i32)  [unwired: 1 in, 1 out]
          n239 = To Quad Integer(1:w1940) -> (0:w1938:i64)
        }
        frame "I16" {
          n240 = Variant To Data(type=i16 0, Variant=w1945) -> (data=w1944:i16)  [unwired: 1 in, 1 out]
          n241 = To Quad Integer(1:w1944) -> (0:w1942:i64)
        }
        frame "I8" {
          n242 = Variant To Data(type=i8 0, Variant=w1949) -> (data=w1948:i8)  [unwired: 1 in, 1 out]
          n243 = To Quad Integer(1:w1948) -> (0:w1946:i64)
        }
        frame "Double Float" {
          n244 = Variant To Data(type=0.0, Variant=w1953) -> (data=w1952:dbl)  [unwired: 1 in, 1 out]
          n245 = Type Cast(type=w1950, x=w1952) -> (*(type *) &x=w1951:i64)
        }
      }
      n246 = case shown="\"Double Float\"" w1858 {
        tunnel: [_ w1916 w1918 w1922 w1926 w1931] -> w1856
        tunnel: w1857 -> [_ w1917 w1921 w1925 w1929 w1933]
        tunnel: [TRUE _ _ _ _ _] -> w1855
        tunnel: w1849 -> [_ w1915 _ _ _ w1930]
        frame "Invalid Type", "Void", Default {
        }
        frame "I64" {
          n247 = Variant To Data(type=w1915, Variant=w1917) -> (data=w1916:i64)  [unwired: 1 in, 1 out]
        }
        frame "I32" {
          n248 = Variant To Data(type=0, Variant=w1921) -> (data=w1920:i32)  [unwired: 1 in, 1 out]
          n249 = To Quad Integer(1:w1920) -> (0:w1918:i64)
        }
        frame "I16" {
          n250 = Variant To Data(type=i16 0, Variant=w1925) -> (data=w1924:i16)  [unwired: 1 in, 1 out]
          n251 = To Quad Integer(1:w1924) -> (0:w1922:i64)
        }
        frame "I8" {
          n252 = Variant To Data(type=i8 0, Variant=w1929) -> (data=w1928:i8)  [unwired: 1 in, 1 out]
          n253 = To Quad Integer(1:w1928) -> (0:w1926:i64)
        }
        frame "Double Float" {
          n254 = Variant To Data(type=0.0, Variant=w1933) -> (data=w1932:dbl)  [unwired: 1 in, 1 out]
          n255 = Type Cast(type=w1930, x=w1932) -> (*(type *) &x=w1931:i64)
        }
      }
      n256 = case shown="\"Double Float\"" w1854 {
        tunnel: [_ w1895 w1897 w1901 w1905 w1910] -> w1852
        tunnel: w1853 -> [_ w1896 w1900 w1904 w1908 w1912]
        tunnel: [TRUE _ _ _ _ _] -> w1851
        tunnel: w1849 -> [_ w1894 _ _ _ w1909]
        frame "Invalid Type", "Void", Default {
        }
        frame "I64" {
          n257 = Variant To Data(type=w1894, Variant=w1896) -> (data=w1895:i64)  [unwired: 1 in, 1 out]
        }
        frame "I32" {
          n258 = Variant To Data(type=0, Variant=w1900) -> (data=w1899:i32)  [unwired: 1 in, 1 out]
          n259 = To Quad Integer(1:w1899) -> (0:w1897:i64)
        }
        frame "I16" {
          n260 = Variant To Data(type=i16 0, Variant=w1904) -> (data=w1903:i16)  [unwired: 1 in, 1 out]
          n261 = To Quad Integer(1:w1903) -> (0:w1901:i64)
        }
        frame "I8" {
          n262 = Variant To Data(type=i8 0, Variant=w1908) -> (data=w1907:i8)  [unwired: 1 in, 1 out]
          n263 = To Quad Integer(1:w1907) -> (0:w1905:i64)
        }
        frame "Double Float" {
          n264 = Variant To Data(type=0.0, Variant=w1912) -> (data=w1911:dbl)  [unwired: 1 in, 1 out]
          n265 = Type Cast(type=w1909, x=w1911) -> (*(type *) &x=w1910:i64)
        }
      }
      n266 = Format Into String(format string=w1862, w1861) -> (resulting string=w1871:string)  [unwired: 2 in, 1 out]
      n267 = Format Into String(format string=w1862, w1856) -> (resulting string=w1867:string)  [unwired: 2 in, 1 out]
      n268 = Format Into String(format string=w1862, w1852) -> (resulting string=w1866:string)  [unwired: 2 in, 1 out]
      n269 = Format Into String(format string=w1862, w1847) -> (resulting string=w1870:string)  [unwired: 2 in, 1 out]
      n270 = Not(x=w1855) -> (.not. x?=w1868:bool)
      n271 = Not(x=w1851) -> (.not. x?=w1869:bool)
      n272 = call "SLSC Convert Items - Min_Max to String.vi"("minimum"=w1867, "maximum"=w1866, "min?"=w1868, "max?"=w1869) -> ("minimum out"=w1864:string, "maximum out"=w1863:string, "minmax string"=w1865:string)  [unwired: 9 in]
    }
    frame "Bool", "Boolean" {
      n273 = Variant To Data(type=FALSE, Variant=w1959) -> (data=w1962:bool, error out=w1961:errorcluster)  [unwired: 1 in]
      n274 = Variant To Data(type=FALSE, Variant=w1966) -> (data=w1963:bool, error out=w1965:errorcluster)  [unwired: 1 in]
      n275 = case shown="Error" w1961 {
        selector: w1961 -> [_ w1979]
        tunnel: w1959 -> [_ w1975]
        tunnel: [w1974 w1980] -> w1956
        tunnel: w1962 -> [w1974 _]
        frame No Error {
        }
        frame Error {
          w1981 = u16 0 items=[""] ("Ring")
          n276 = Variant To Data(error in=w1979, type=w1981, Variant=w1975) -> (data=w1976:u16, error out=w1978:errorcluster)
          n277 = case shown="Error" w1978 {
            selector: w1978 -> [_ w1987]
            tunnel: [w1982 w1984] -> w1977
            tunnel: w1976 -> [w1982 _]
            tunnel: w1975 -> [_ w1986]
            frame No Error {
            }
            frame Error {
              n278 = Variant To Data(error in=w1987, type=0.0, Variant=w1986) -> (data=w1983:dbl, error out=w1985:errorcluster)
              n279 = case shown="Error" w1985 {
                tunnel: w1986 -> [_ w1991]
                tunnel: [w1989 w1990] -> w1984
                tunnel: w1983 -> [w1989 _]
                frame No Error {
                }
                frame Error {
                  n280 = Variant To Data(type=u32 0, Variant=w1991) -> (data=w1990:u32)  [unwired: 1 in, 1 out]
                }
              }
            }
          }
          n281 = Not Equal To 0?(x=w1977) -> (x != 0?=w1980:bool)
        }
      }
      n282 = case shown="Error" w1965 {
        selector: w1965 -> [_ w1998]
        tunnel: w1966 -> [_ w1994]
        tunnel: [w1993 w1999] -> w1964
        tunnel: w1963 -> [w1993 _]
        frame No Error {
        }
        frame Error {
          w2000 = u16 0 items=[""] ("Ring")
          n283 = Variant To Data(error in=w1998, type=w2000, Variant=w1994) -> (data=w1995:u16, error out=w1997:errorcluster)
          n284 = case shown="Error" w1997 {
            selector: w1997 -> [_ w2006]
            tunnel: [w2001 w2003] -> w1996
            tunnel: w1995 -> [w2001 _]
            tunnel: w1994 -> [_ w2005]
            frame No Error {
            }
            frame Error {
              n285 = Variant To Data(error in=w2006, type=0.0, Variant=w2005) -> (data=w2002:dbl, error out=w2004:errorcluster)
              n286 = case shown="Error" w2004 {
                tunnel: w2005 -> [_ w2010]
                tunnel: [w2008 w2009] -> w2003
                tunnel: w2002 -> [w2008 _]
                frame No Error {
                }
                frame Error {
                  n287 = Variant To Data(type=u32 0, Variant=w2010) -> (data=w2009:u32)  [unwired: 1 in, 1 out]
                }
              }
            }
          }
          n288 = Not Equal To 0?(x=w1996) -> (x != 0?=w1999:bool)
        }
      }
      n289 = Boolean To (0,1)(Boolean=w1964) -> (0, 1=w1968:i16)
      n290 = Select(t="True" ("data string"), s=w1964, f="False" ("data string")) -> (s? t:f=w1971:string)
      n291 = Select(t="True" ("data string"), s=w1956, f="False" ("data string")) -> (s? t:f=w1955:string)
      n292 = Number To Decimal String(number=w1968) -> (decimal integer string=w1967:string)  [unwired: 1 in]
    }
    frame "String" {
      w2014 = "" ("data string")
      n293 = Variant To Data(type=w2014, Variant=w2016) -> (data=w2015:string)  [unwired: 1 in, 1 out]
      n294 = Variant To Data(type=w2014, Variant=w2013) -> (data=w2012:string)  [unwired: 1 in, 1 out]
    }
  }
  "enum_range" <- w14
  "Output data type" <- w10
  "string data value" <- w3
  "string min" <- w6
  "string max" <- w5
  "Option" <- w4
  "string data reset value" <- w1
